vi "Check valid path.vi"(11 "Path":path) -> (3 "valid path":bool)   [LabVIEW 2017]
uses:
  <vilib>/regexp/Match Regular Expression.xnode
panel:
  out "offset past match":i32
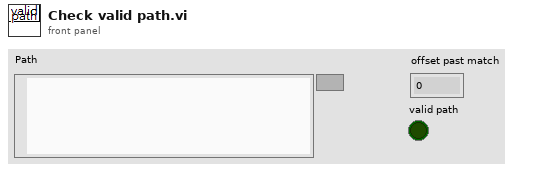
[diagram p1: front panel]
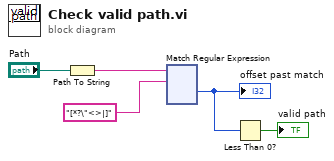
[diagram p0: block diagram]
diagram:
  n1 = Path To String(path="Path") -> (string=w4:string)
  n2 = xnode "Match Regular Expression"("input string"=w4, "regular expression"="[*?\"<>|]") -> ("offset past match"=w2:i32)  [unwired: 4 in, 4 out]
  "offset past match" <- w2
  n3 = Less Than 0?(x=w2) -> (x < 0?=→"valid path":bool)
